vi "Create All Message Queues.vi"(8 "error in (no error)":errorcluster) -> (0 "error out":errorcluster, 3 "Message Queues out":T1)   [LabVIEW 2017, in "CL_G3_BuilderApplicationLayer.lvlib" / "Message Queue.lvlib"]
doc: "This VI creates and initializes all the message queues for your application. If your application requires more than one message queue, right-click the \"Message Queues\" constant above and select Open Type Def. Add the new Message Queue(s) to the type definition, then initialize them in this VI."
uses:
  Message Queue.lvlib
  All Message Queues.ctl
  Message Cluster.ctl
  Enqueue Message (Single).vi
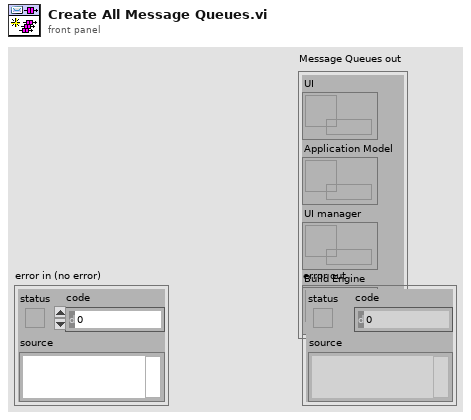
[diagram p1: front panel]
types:
  T1 = typedef "CL_G3_BuilderApplicationLayer.lvlib/Message Queue.lvlib/All Message Queues.ctl" = cluster{"UI":refnum<queue>, "Application Model":refnum<queue>, "UI manager":refnum<queue>, "Build Engine":refnum<queue>}
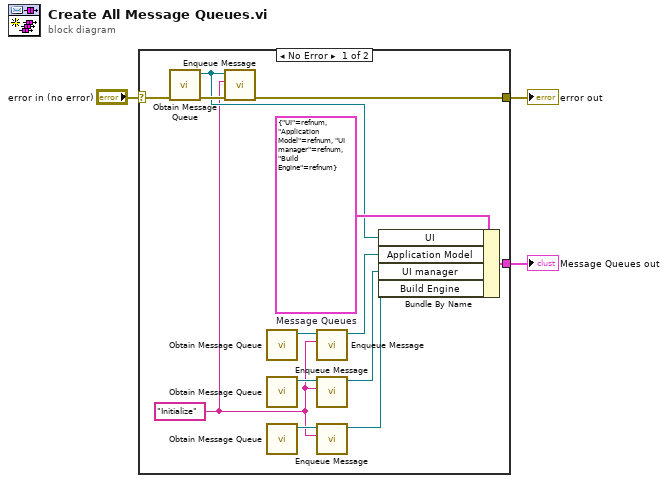
[diagram p0: block diagram]
diagram:
  n1 = case shown="No Error" "error in (no error)" {
    selector: "error in (no error)" -> [w13 w17]
    tunnel: [w16 w17] -> w3
    tunnel: [w14 _] -> w2
    frame No Error {
      w7 = "Initialize" ("Message")
      w15 = T1 {"UI"=refnum, "Application Model"=refnum, "UI manager"=refnum, "Build Engine"=refnum}  # Message Queues
      n2 = call "Obtain Message Queue.vi"("error in (no error)"=w13) -> ("error out"=w12:errorcluster, "Message Queue"=w11:refnum<queue>)  [unwired: 9 in]
      n3 = call-poly "Enqueue Message.vi"("error in (no error)"=w12, "Message"=w7, "Message Queue"=w11) -> ("error out"=w16:errorcluster)  [unwired: 7 in, 1 out]
      n4 = call "Obtain Message Queue.vi"() -> ("Message Queue"=w10:refnum<queue>)  [unwired: 10 in, 1 out]
      n5 = call "Obtain Message Queue.vi"() -> ("Message Queue"=w9:refnum<queue>)  [unwired: 10 in, 1 out]
      n6 = call "Obtain Message Queue.vi"() -> ("Message Queue"=w8:refnum<queue>)  [unwired: 10 in, 1 out]
      n7 = call-poly "Enqueue Message.vi"("Message"=w7, "Message Queue"=w10) -> ("dup Message Queue"=w6:refnum<queue>)  [unwired: 8 in, 1 out]
      n8 = call-poly "Enqueue Message.vi"("Message"=w7, "Message Queue"=w9) -> ("dup Message Queue"=w5:refnum<queue>)  [unwired: 8 in, 1 out]
      n9 = call-poly "Enqueue Message.vi"("Message"=w7, "Message Queue"=w8) -> ("dup Message Queue"=w4:refnum<queue>)  [unwired: 8 in, 1 out]
      n10 = Bundle By Name(cluster=w15, "UI"=w11, "Application Model"=w6, "UI manager"=w5, "Build Engine"=w4) -> (w14:T1)
    }
    frame Error {
    }
  }
  "Message Queues out" <- w2
  "error out" <- w3
